vi "Data_Collection_GCFS.vi"(5 "Properties":T1[](array[typedef]), 7 "Groups":string, 8 "error in":errorcluster, 9 "Droplet num":bool, 10 "Image":T2, 11 "Session":T3) -> (0 "error out":errorcluster, 1 "date/time string":string, 2 "Image Out":T2, 3 "Temperature":dbl)   [LabVIEW 2024]
uses:
  <vilib>/userDefined/High Color/IMAQdx.ctl
  <vilib>/vision/Image Controls.llb/IMAQ Image.ctl
  <vilib>/vision/Image Controls.llb/Overlay Property.ctl
  <vilib>/vision/driver/IMAQdx.llb/IMAQdx Buffer Number Mode.ctl
  <vilib>/vision/driver/NI_Vision_Acquisition_Software.lvlib
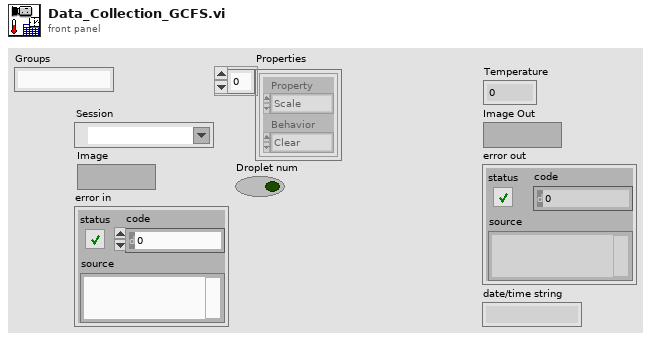
[diagram p1: front panel]
types:
  T1 = typedef "Overlay Property.ctl" = cluster{"Property":enum32{"Scale", "Shift", "Rotate", "Symmetry"}, "Behavior":enum32{"Clear", "Keep", "Transform"}}
  T2 = typedef "IMAQ Image.ctl" = refnum<image>
  T3 = typedef "IMAQdx.ctl" = refnum<k21>
  T4 = typedef "NI_Vision_Acquisition_Software.lvlib/IMAQdx Buffer Number Mode.ctl" = enum32{"Next", "Last", "Buffer Number", "Every", "Last New"}
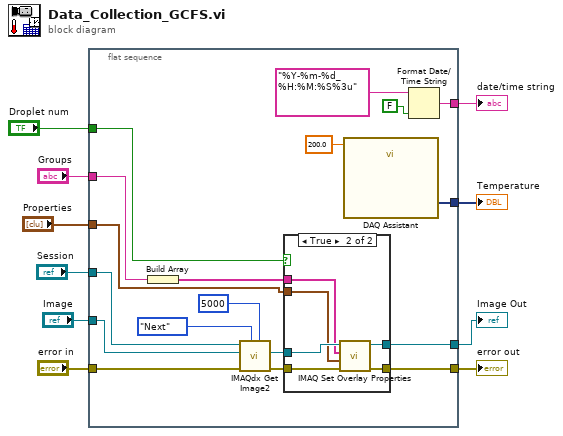
[diagram p0: block diagram]
diagram:
  n1 = flat-sequence {
    tunnel: "Session" -> [w27]
    tunnel: "Image" -> [w26]
    tunnel: "error in" -> [w24]
    tunnel: [w17] -> w6
    tunnel: [w16] -> w7
    tunnel: [w21] -> w5
    tunnel: [w19] -> w4
    tunnel: "Properties" -> [w14]
    tunnel: "Droplet num" -> [w13]
    tunnel: "Groups" -> [w12]
    frame #0 {
      n2 = Build Array(w12) -> (w11:string[])
      n3 = call <vilib>:"IMAQdx Get Image2.vi"("Timeout (ms)"=5000, "Buffer Number Mode (Next)"=IMAQdx_Buffer_Number_Mode."Next", "error in"=w24, "Image In"=w26, "Session In"=w27) -> ("error out"=w18:errorcluster, "Image Out"=w15:T2)  [unwired: 3 in, 2 out]
      n4 = case shown="True" w13 {
        tunnel: [w29 w33] -> w17
        tunnel: w18 -> [w29 w34]
        tunnel: [w30 w36] -> w16
        tunnel: w15 -> [w30 w35]
        tunnel: w14 -> [_ w32]
        tunnel: w11 -> [_ w31]
        frame False {
        }
        frame True {
          n5 = call "IMAQ Set Overlay Properties"("Image"=w35, "Groups"=w31, "Properties"=w32, "error in (no error)"=w34) -> ("Image Out"=w36:T2, "error out"=w33:errorcluster)  [unwired: 4 in]
        }
      }
      n6 = call "DAQ Assistant"("timeout (s)"=200.0) -> ("data"=w19:dynamicdata)  [unwired: 16 in, 2 out]
      n7 = Format Date/Time String(time format string (%c)="%Y-%m-%d_%H:%M:%S%3u", UTC format=FALSE) -> (date/time string=w21:string)  [unwired: 1 in]
    }
  }
  "Image Out" <- w7
  "error out" <- w6
  "date/time string" <- w5
  "Temperature" <- w4
